vi "Communication - Iteration Data (FGV).vi"(7 "Action":T1=enum."Write", 8 "error in (no error)":errorcluster, 11 "Iteration SV":i64[](array[numeric])) -> (0 "error out":errorcluster, 3 "Iteration SV Out":i64[](array[numeric]))   [LabVIEW 2019]
uses:
  Controls/FGV States.ctl
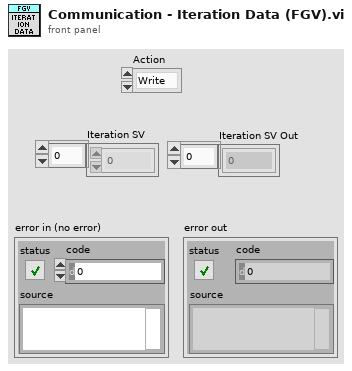
[diagram p1: front panel]
types:
  T1 = typedef "FGV States.ctl" = enum16{"Read", "Write"}
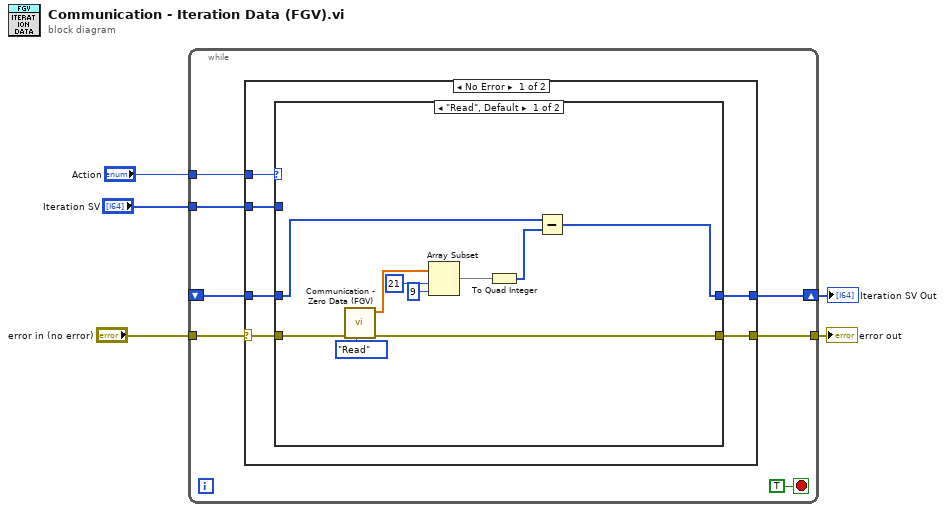
[diagram p0: block diagram]
diagram:
  n1 = while {
    tunnel: "Action" -> [w12]
    tunnel: "Iteration SV" -> [w10]
    shift-right: [w11] -> w3
    shift-left: _ -> [w9]
    tunnel: "error in (no error)" -> [w7]
    tunnel: [w6] -> w1
    stop <- TRUE stop-if-true
    n2 = case shown="No Error" w7 {
      selector: w7 -> [w13 w31]
      tunnel: w12 -> [w18 _]
      tunnel: [w17 w32] -> w11
      tunnel: w10 -> [w16 _]
      tunnel: w9 -> [w15 w32]
      tunnel: [w14 w31] -> w6
      frame No Error {
        n3 = case shown="\"Read\", Default" w18 {
          tunnel: [w19 w30] -> w17
          tunnel: w16 -> [_ w30]
          tunnel: w15 -> [w21 _]
          tunnel: [w27 w29] -> w14
          tunnel: w13 -> [w26 w29]
          frame "Read", Default {
            n4 = call "Communication - Zero Data (FGV).vi"("Action"=FGV_States."Read", "error in (no error)"=w26) -> ("error out"=w27:errorcluster, "Zero Out"=w25:dbl[])  [unwired: 8 in]
            n5 = Array Subset(array=w25, index=21, length=9) -> (w22:dbl[])
            n6 = To Quad Integer(1:w22) -> (0:w20:i64[])
            n7 = Subtract(x=w21, y=w20) -> (x-y=w19:i64[])
          }
          frame "Write" {
          }
        }
      }
      frame Error {
      }
    }
  }
  "Iteration SV Out" <- w3
  "error out" <- w1
